vi "Vision Time AE.vi"() -> (2 "Vision Talking?":bool)   [LabVIEW 2025]
uses:
  <vilib>/Rock Robotics/Network Tables/NT Read Number.vi
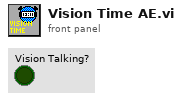
[diagram p1: front panel]
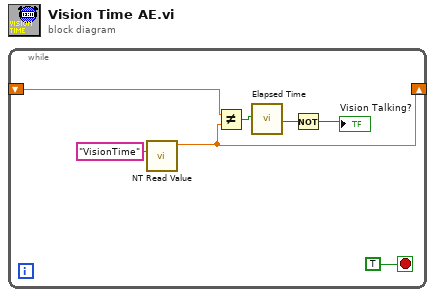
[diagram p0: block diagram]
diagram:
  n1 = while {
    shift-right: [w4] -> _
    shift-left: _ -> [w5]
    stop <- TRUE stop-if-true
    n2 = call-poly <vilib>:"NT Read Value.vi"("name"="VisionTime" ("Name")) -> ("value"=w4:dbl)  [unwired: 8 in, 2 out]
    n3 = Not Equal?(x=w5, y=w4) -> (x != y?=w3:bool)
    n4 = call "Elapsed Time"("Reset"=w3) -> ("Time has Elapsed"=w2:bool)  [unwired: 11 in, 7 out]
    n5 = Not(x=w2) -> (.not. x?=→"Vision Talking?":bool)
  }
